vi "界面UI.vi"() -> ()   [LabVIEW 2016, in "德润DR803L超标留样.lvlib"]
uses:
  <vilib>/Utility/miscctls.llb/LVPointTypeDef.ctl
  <vilib>/Utility/config.llb/NI_LVConfig.lvlib
  <vilib>/ptbypt/NI_PtbyPt.lvlib
panel:
  in  "单步控制":bool
  in  "设置":bool
  out "采样器进程 2":T1(ring)
  out "单次采样量":u16
  out "留样模式":T2(ring)
  out "门状态":enum16{"门开", "门关"}(ring)
  out "报警状态":enum16{"无报警", "缺水报警"}(ring)
  out "仪器时间":timestamp format="%<%Y/%m/%d %H:%M:%S>T"
  out "当前瓶号":u16
  out "采样器状态":enum16{"停止", "运行"}(ring)
  out "采样器进程":i32(listbox)
  out "流程中":bool
  in  "停止流程":bool
  in  "启动流程":bool
  in  "修改门禁密码":bool
  in  "远程复位":bool
  in  "远程留样":bool
  out "Registers":u16[](array[numeric])
  in  "采样启动":bool
  in  "停止命令":bool
  in  "切换采样器状态":bool
  in  "时间校准":bool
  out "通讯":bool
  # "只在待机时启动有效"
  # "德润DR803L超标留样"
  # "只在待机时启动有效"
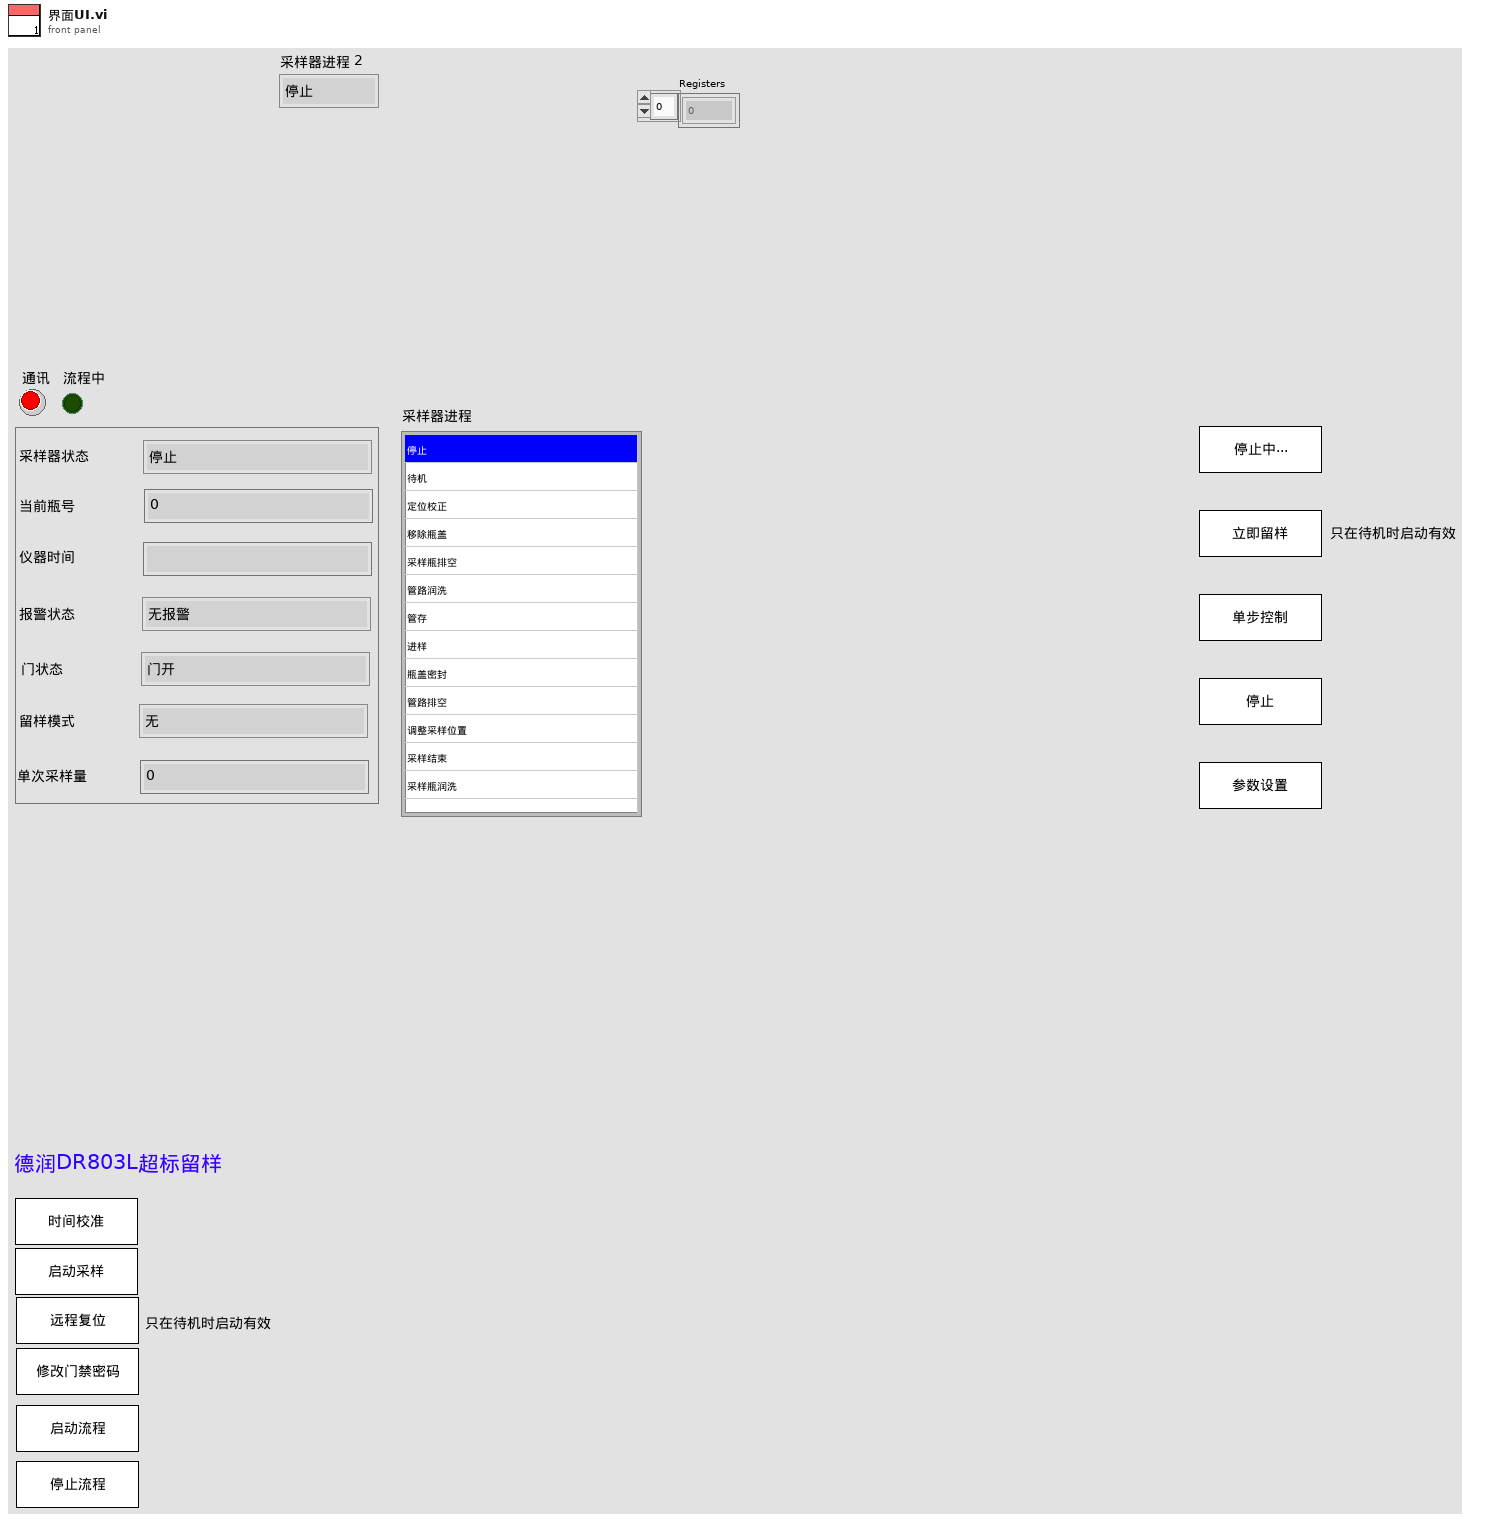
[diagram p1: front panel]
types:
  T1 = enum16{"停止", "待机", "定位校正", "移除瓶盖", "采样瓶排空", "管路润洗", "管存", "进样", "瓶盖密封", "管路排空", "调整采样位置", "采样结束", "采样瓶润洗", "瓶润洗排空"}
  T2 = enum16{"无", "定时留样", "时间等比例", "超标留样", "同步留样", "外控留样"}
  T3 = cluster{"STEP":enum16{"open", "read", "write", "write single", "close"}, "starting address":u16, "value":u16}
  T4 = typedef "LVPointTypeDef.ctl" = cluster{"Horizontal":i16, "Vertical":i16}
  T5 = typedef "NI_LVConfig.lvlib/Config Data RefNum.ctl" = refnum<k1>
  T6 = enum16{"open", "read", "write", "write single", "close"}
  T7 = typedef "LVDateTimeRec.ctl" = cluster{"秒数的小数部分":dbl, "秒":i32, "分":i32, "时":i32, "日":i32, "月":i32, "年":i32, "天数（周）":i32, "天数（年）":i32, "DST":i32}
  T8 = enum32{"Bad", "Idle", "Run top level", "Running"}
  T9 = cluster{"采样器状态":enum16{"停止", "运行"}, "当前留样瓶编号":u16, "报警状态":enum16{"无报警", "缺水报警"}, "超标信号":enum16{"无信号", "超标信号"}, "采样器进程":enum16{"停止", "待机", "定位校正", "移除瓶盖", "采样瓶排空", "管路润洗", "管存", "进样", "瓶盖密封", "管路排空", "调整采样位置", "采样结束", "采样瓶润洗", "瓶润洗排空"}, "版本号":string, "同步信号":enum16{"无信号", "同步信号"}, "外控信号":enum16{"无信号", "外控信号"}, "门状态":enum16{"门开", "门关"}, "当前瓶号":u16, "工作状态":enum16{"停止", "采样中"}, "留样模式":enum16{"无", "定时留样", "时间等比例", "超标留样", "同步留样", "外控留样"}, "立即留样":enum16{"无", "远程留样"}, "采样方式":enum16{"单采", "双重"}, "仪器时间":timestamp, "单次采样量":u16, "时间等比采样采样间隔":u16, "排空命令":u16, "远程复位":u16, "门禁密码":u16}
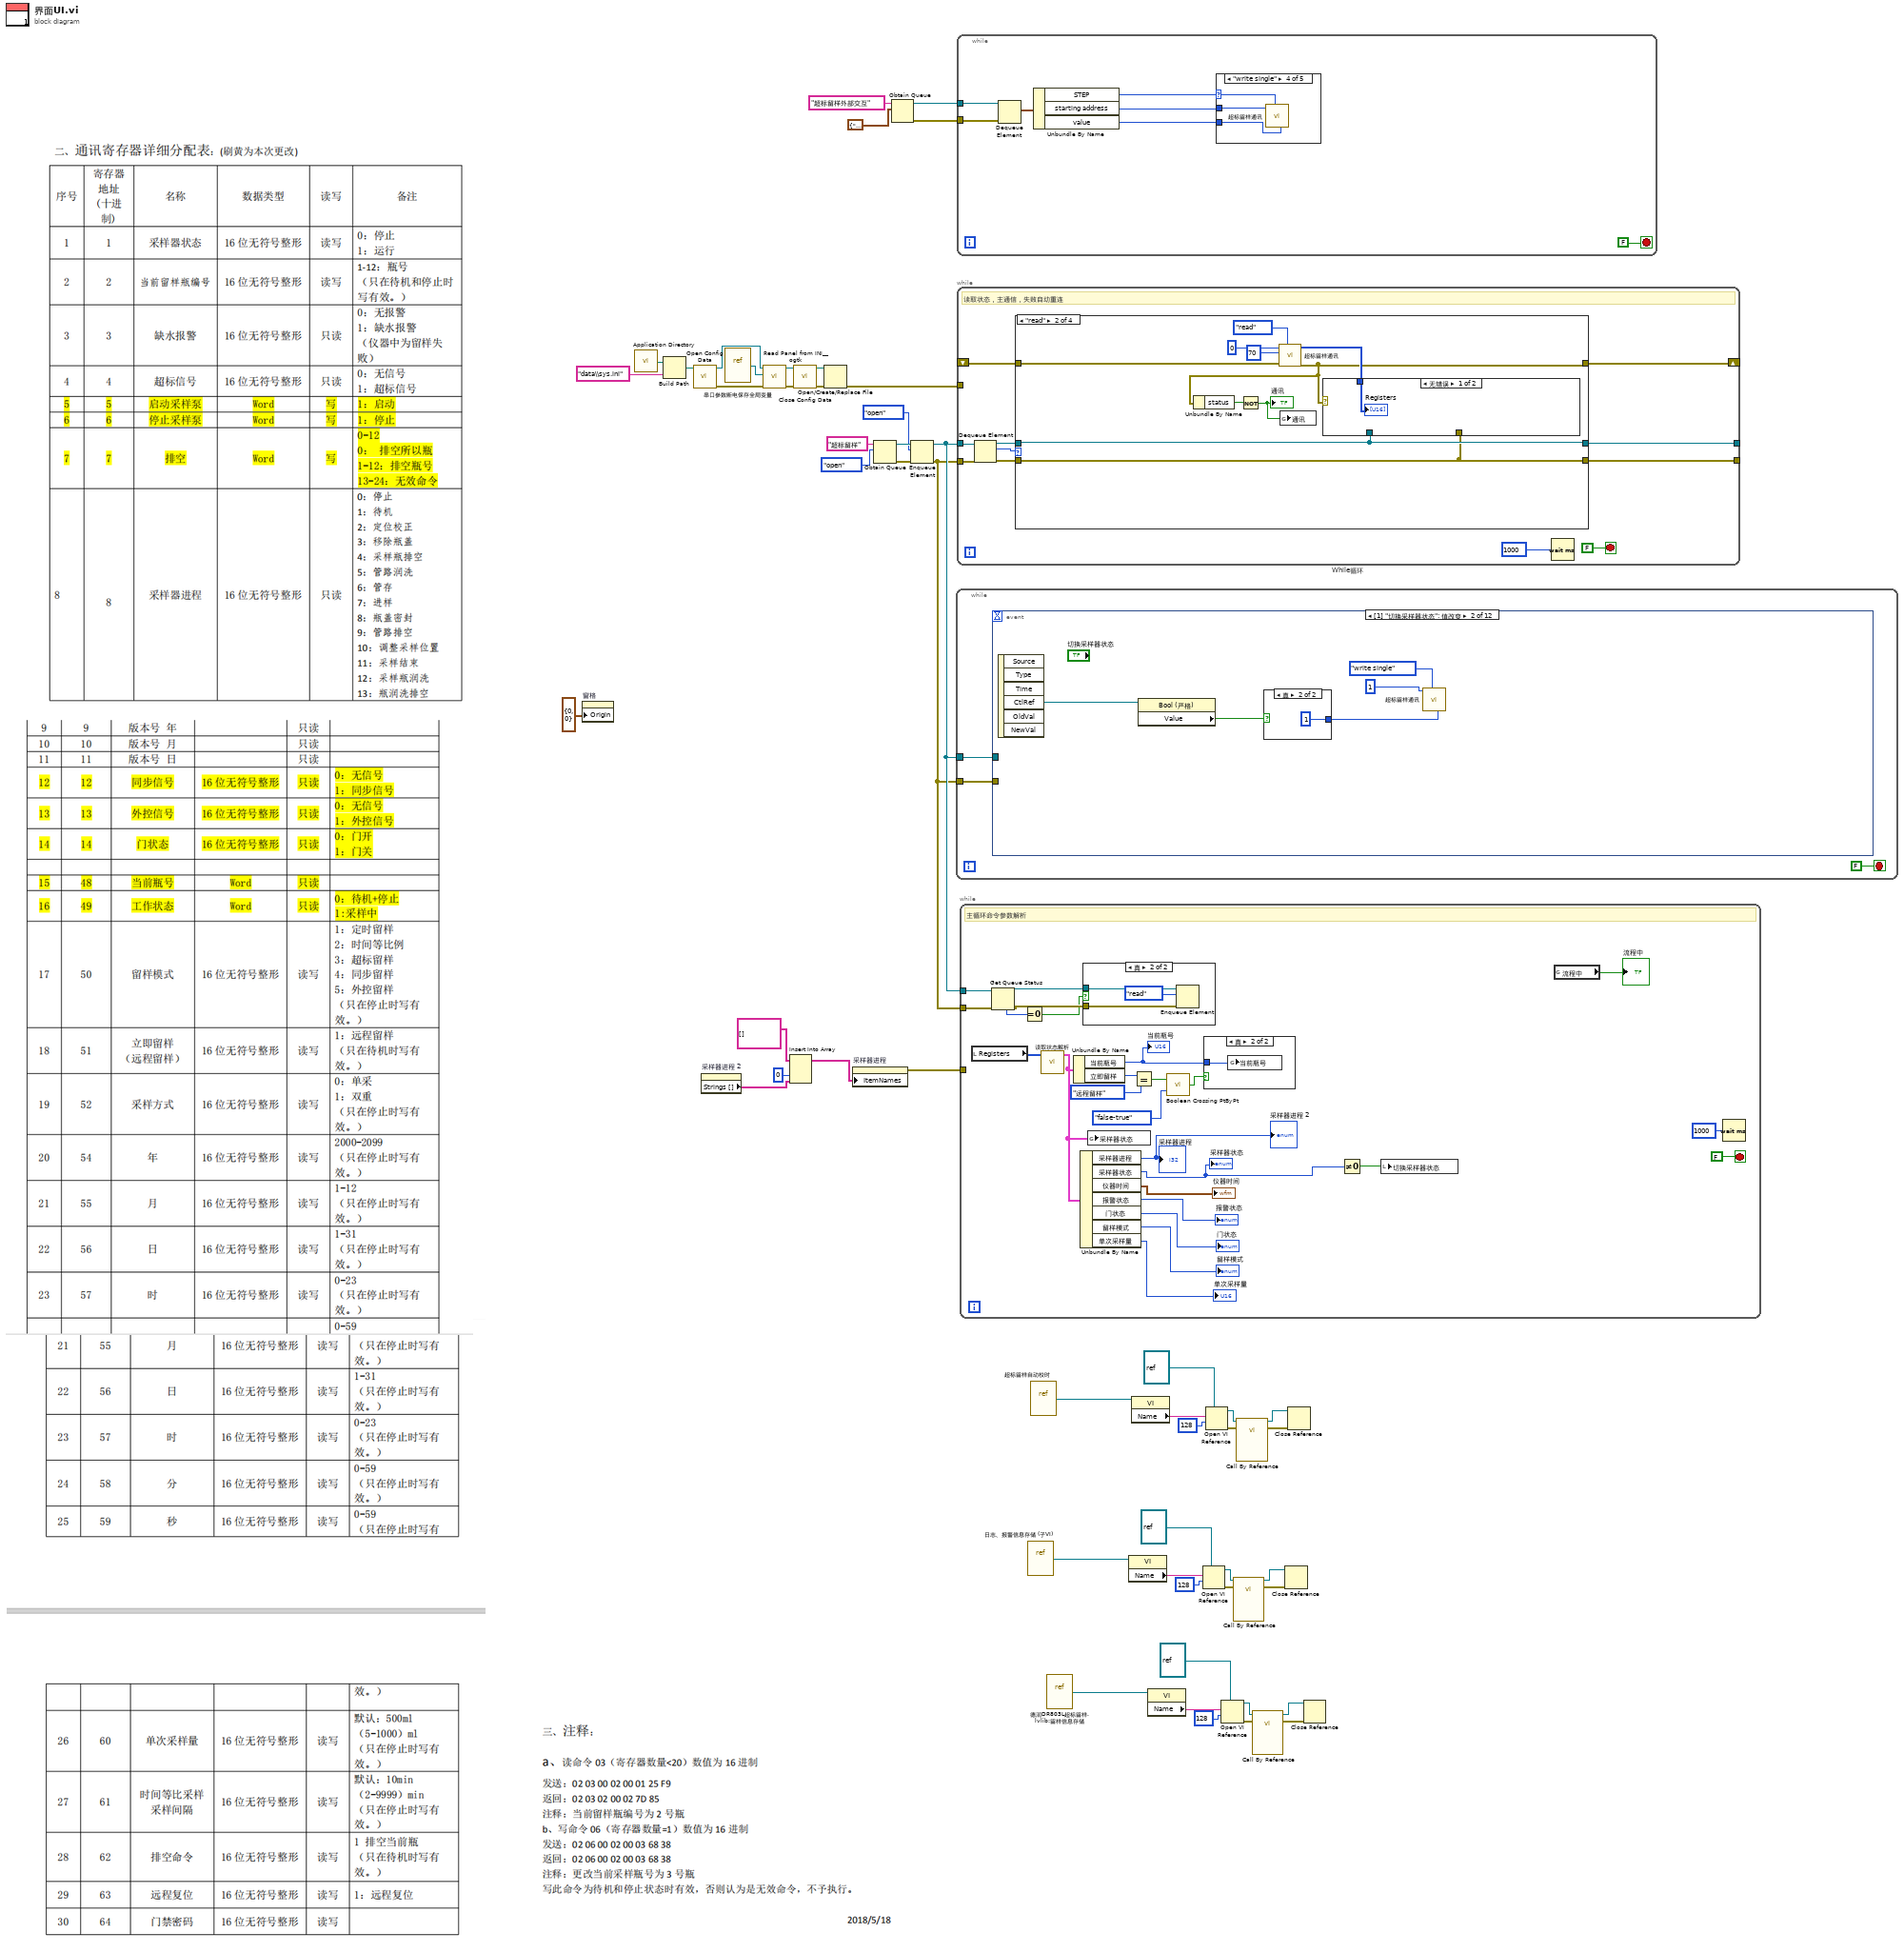
[diagram p0: block diagram]
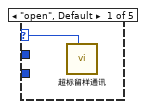
[diagram p2: hidden frame]
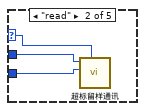
[diagram p3: hidden frame]
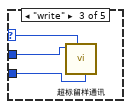
[diagram p4: hidden frame]
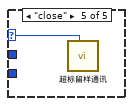
[diagram p5: hidden frame]
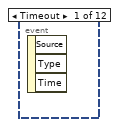
[diagram p6: hidden frame]
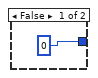
[diagram p7: hidden frame]
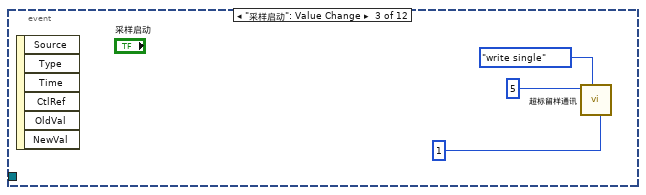
[diagram p8: hidden frame]
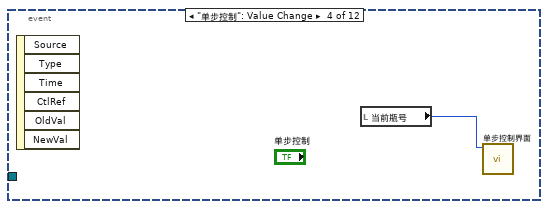
[diagram p9: hidden frame]
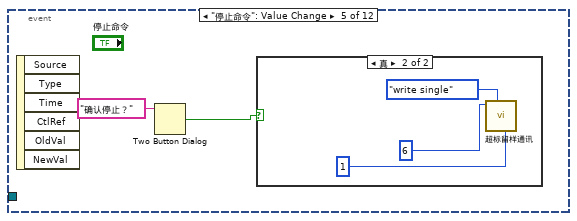
[diagram p10: hidden frame]
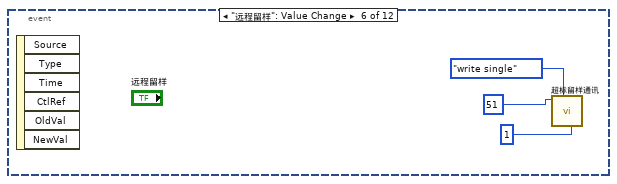
[diagram p12: hidden frame]
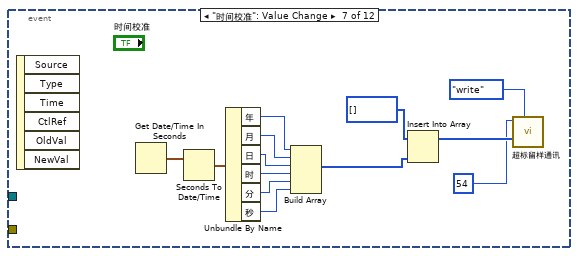
[diagram p13: hidden frame]
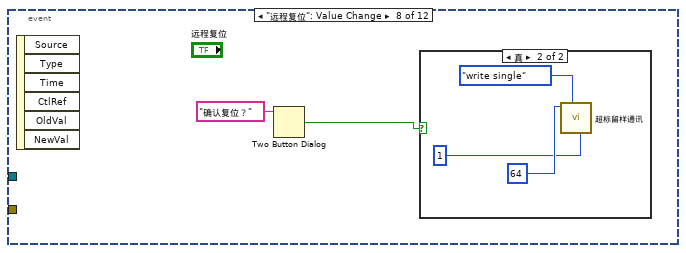
[diagram p14: hidden frame]
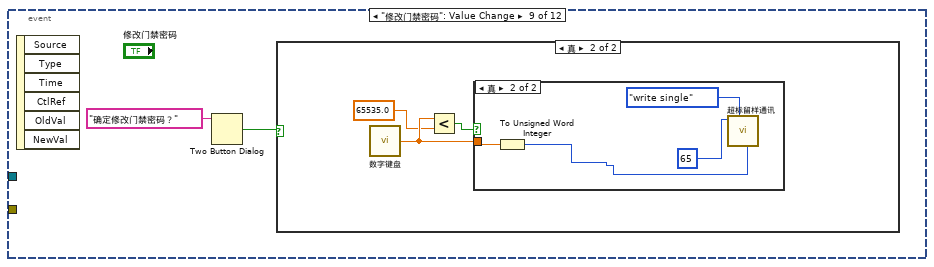
[diagram p16: hidden frame]
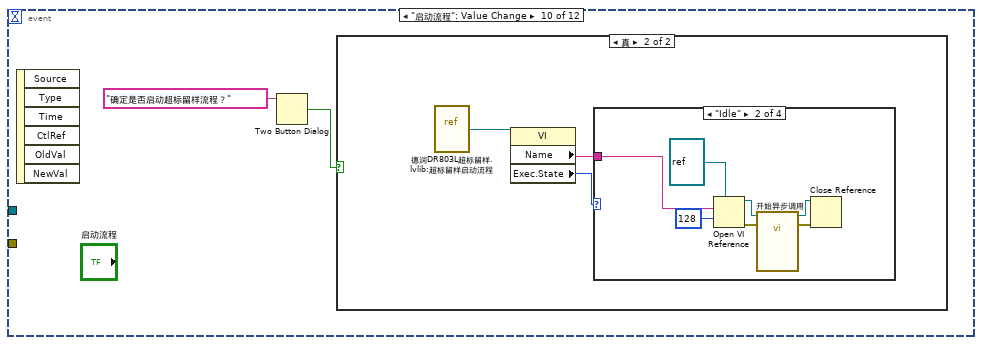
[diagram p19: hidden frame]
diagram:
  n1 = property on="窗格" class="Pane"("Origin"=T4 {"Horizontal"=0, "Vertical"=0} ("原点")) -> ()  [unwired: 2 in, 2 out]
  n2 = call <vilib>:"Application Directory.vi"() -> ("Application Directory"=w44:path)
  n3 = Build Path(base path=w44, name or relative path="data\\sys.ini" ("名称或相对路径")) -> (appended path=w42:path)
  n4 = call <vilib>:"Open Config Data.vi"("configuration file path"=w42) -> ("error out"=w38:errorcluster, "refnum"=w41:T5)  [unwired: 8 in, 1 out]
  n5 = property on="采样器进程 2" class="Enum (严格)"() -> ("Strings []"=w9:string[])  [unwired: 2 in, 2 out]
  n6 = vi-ref "串口参数断电保存全局变量.vi"() -> (w40:refnum<vi>)
  n7 = call <userlib>:"Read Panel from INI__ogtk.vi"("error in (no error)"=w38, "VI ref"=w40, "refnum"=w41) -> ("error out"=w37:errorcluster, "refnum out"=w39:T5)  [unwired: 7 in]
  n8 = Insert Into Array(array=string[][] [] ("字符串[]"), index (col)=0 ("禁用的索引 (列)"), new element=w9) -> (w11:string[][])  [unwired: 1 in]
  n9 = call <vilib>:"Close Config Data.vi"("error in (no error)"=w37, "refnum"=w39) -> ("error out"=w36:errorcluster, "file path"=w35:path)  [unwired: 8 in]
  n10 = Open/Create/Replace File(file path (use dialog)=w35, error in=w36) -> (error out=w34:errorcluster)  [unwired: 4 in, 2 out]
  n11 = property on="采样器进程" class="MCListbox (严格)"("ItemNames"=w11) -> (error out=w10:errorcluster)  [unwired: 2 in, 1 out]
  n12 = Obtain Queue(name (unnamed)="超标留样" ("名称（未命名）"), element data type=enum16{"open", "read", "write", "close"}."open") -> (queue out=w50:refnum<queue>, error out=w49:errorcluster)  [unwired: 3 in, 1 out]
  n13 = Obtain Queue(name (unnamed)="超标留样外部交互" ("名称（未命名）"), element data type=T3 {"STEP"=enum."write single", "starting address"=0, "value"=0}) -> (queue out=w31:refnum<queue>, error out=w30:errorcluster)  [unwired: 3 in, 1 out]
  n14 = Enqueue Element(queue=w50, element=enum16{"open", "read", "write", "close"}."open", error in (no error)=w49) -> (queue out=w47:refnum<queue>, error out=w46:errorcluster)  [unwired: 1 in, 1 out]
  n15 = while {
    tunnel: w47 -> [w54]
    tunnel: w46 -> [w53]
    stop <- FALSE stop-if-true
    n16 = event shown="[1] \"切换采样器状态\": 值改变" {
      selector: _ -> [_ _ _ _ _ _ _ _ _ _ _ _]
      dyn-events: _ -> [_ _ _ _ _ _ _ _ _ _ _ _]
      timeout: _ -> [_ _ _ _ _ _ _ _ _ _ _ _]
      tunnel: w54 -> [_ _ _ _ _ _ _ _ _ _ _ _]
      tunnel: w53 -> [_ _ _ _ _ _ _ _ _ _ _ _]
      event Timeout {
        n17 = event-data() -> ()  [unwired: 1 in, 3 out]
      }
      event "切换采样器状态": Value Change {
        n18 = event-data() -> ("CtlRef"=w60:refnum<vi>)  [unwired: 1 in, 5 out]
        n19 = property class="Bool (严格)"(reference=w60) -> ("Value"=w59:bool)  [unwired: 1 in, 2 out]
        n20 = case shown="真" w59 {
          tunnel: [u16 0 ("索引") u16 1 ("索引")] -> w56
          frame False {
          }
          frame True {
          }
        }
        n21 = call "超标留样通讯.vi"("value"=w56, "STEP"=T6."write single", "starting address"=1 ("索引")) -> ()  [unwired: 6 in, 3 out]
      }
      event "采样启动": Value Change {
        n22 = event-data() -> ()  [unwired: 1 in, 6 out]
        n23 = call "超标留样通讯.vi"("value"=u16 1 ("新元素/子数组"), "STEP"=T6."write single", "starting address"=5 ("索引")) -> ()  [unwired: 6 in, 3 out]
      }
      event "单步控制": Value Change {
        n24 = event-data() -> ()  [unwired: 1 in, 6 out]
        n25 = local read "当前瓶号"() -> (w66:u16)
        n26 = call "单步控制界面.vi"("当前瓶号"=w66) -> ()  [unwired: 11 in]
      }
      event "停止命令": Value Change {
        n27 = event-data() -> ()  [unwired: 1 in, 6 out]
        n28 = Two Button Dialog(message="确认停止？" ("消息")) -> (T button?=w67:bool)  [unwired: 2 in]
        n29 = case shown="真" w67 {
          frame False {
          }
          frame True {
            n30 = call "超标留样通讯.vi"("value"=u16 1 ("新元素/子数组"), "STEP"=T6."write single", "starting address"=6 ("索引")) -> ()  [unwired: 6 in, 3 out]
          }
        }
      }
      event "远程留样": Value Change {
        n31 = event-data() -> ()  [unwired: 1 in, 6 out]
        n32 = call "超标留样通讯.vi"("value"=u16 1 ("新元素/子数组"), "STEP"=T6."write single", "starting address"=51 ("索引")) -> ()  [unwired: 6 in, 3 out]
      }
      event "时间校准": Value Change {
        n33 = event-data() -> ()  [unwired: 1 in, 6 out]
        n34 = Get Date/Time In Seconds() -> (seconds since 1Jan1904=w87:timestamp)
        n35 = Seconds To Date/Time(time stamp (now)=w87) -> (date time rec=w86:T7)  [unwired: 1 in]
        n36 = Unbundle By Name(w86) -> ("年"=w83:i32, "月"=w82:i32, "日"=w81:i32, "时"=w80:i32, "分"=w79:i32, "秒"=w78:i32)
        n37 = Build Array(w83, w82, w81, w80, w79, w78) -> (w77:i32[])
        n38 = Insert Into Array(array=u16[] [] ("values"), new element=w77) -> (w84:u16[])  [unwired: 1 in]
        n39 = call "超标留样通讯.vi"("STEP"=T6."write", "values"=w84, "starting address"=54 ("索引")) -> ()  [unwired: 6 in, 3 out]
      }
      event "远程复位": Value Change {
        n40 = event-data() -> ()  [unwired: 1 in, 6 out]
        n41 = Two Button Dialog(message="确认复位？" ("消息")) -> (T button?=w88:bool)  [unwired: 2 in]
        n42 = case shown="真" w88 {
          frame False {
          }
          frame True {
            n43 = call "超标留样通讯.vi"("value"=u16 1 ("新元素/子数组"), "STEP"=T6."write single", "starting address"=64 ("索引")) -> ()  [unwired: 6 in, 3 out]
          }
        }
      }
      event "修改门禁密码": Value Change {
        n44 = event-data() -> ()  [unwired: 1 in, 6 out]
        n45 = Two Button Dialog(message="确定修改门禁密码？" ("消息")) -> (T button?=w93:bool)  [unwired: 2 in]
        n46 = case shown="真" w93 {
          frame False {
          }
          frame True {
            n47 = call "数字键盘.vi"() -> ("NewNumber"=w97:sgl)  [unwired: 1 in]
            n48 = Less?(x=w97, y=sgl 65535.0) -> (x < y?=w95:bool)
            n49 = case shown="真" w95 {
              tunnel: w97 -> [_ w101]
              frame False {
              }
              frame True {
                n50 = To Unsigned Word Integer(number=w101) -> (unsigned 16bit integer=w98:u16)
                n51 = call "超标留样通讯.vi"("value"=w98, "STEP"=T6."write single", "starting address"=65 ("索引")) -> ()  [unwired: 6 in, 3 out]
              }
            }
          }
        }
      }
      event "启动流程": Value Change {
        n52 = event-data() -> ()  [unwired: 1 in, 6 out]
        n53 = Two Button Dialog(message="确定是否启动超标留样流程？" ("消息")) -> (T button?=w102:bool)  [unwired: 2 in]
        n54 = case shown="真" w102 {
          frame False {
          }
          frame True {
            n55 = vi-ref "德润DR803L超标留样.lvlib:超标留样启动流程.vi"() -> (w104:refnum<vi>)
            n56 = property class="VI"(reference=w104) -> ("Name"=w105:string, "Exec.State"=w106:T8)  [unwired: 1 in, 2 out]
            n57 = case shown="\"Idle\"" w106 {
              tunnel: w105 -> [_ w109 _ _]
              frame "Bad", Default {
              }
              frame "Idle" {
                n58 = Open VI Reference(type specifier VI Refnum (for type only)=refnum<vi> refnum ("类型说明符VI引用句柄（仅用于类型）"), vi path=w109, options=128 ("选项")) -> (vi reference=w113:refnum<vi>, error out=w108:errorcluster)  [unwired: 3 in]
                n59 = call-by-ref "开始异步调用"(reference=w113, error in=w108) -> (reference out=w112:refnum<vi>, error out=w107:errorcluster)  [unwired: 12 in]
                n60 = Close Reference(reference=w112, error in (no error)=w107) -> ()  [unwired: 1 out]
              }
              frame "Run top level" {
              }
              frame "Running" {
              }
            }
          }
        }
      }
      event "停止流程": Value Change {
        n61 = event-data() -> ()  [unwired: 1 in, 6 out]
        n62 = Two Button Dialog(message="确定是否停止超标留样流程并排空当前瓶？" ("消息")) -> (T button?=w114:bool)  [unwired: 2 in]
        n63 = case shown="真" w114 {
          frame False {
          }
          frame True {
            n64 = Obtain Notifier(name (unnamed)="超标留样流程" ("名称（未命名）"), notification data type=FALSE ("采样完成")) -> (notifier out=w127:refnum<notifier>, error out=w126:errorcluster)  [unwired: 2 in, 1 out]
            n65 = Send Notification(notification=TRUE ("通知"), notifier=w127, error in (no error)=w126) -> (notifier out=w124:refnum<notifier>, error out=w123:errorcluster)
            n66 = call "超标留样通讯.vi"("value"=u16 1 ("新元素/子数组"), "STEP"=T6."write single", "starting address"=6 ("索引")) -> ("error out"=w116:errorcluster)  [unwired: 6 in, 2 out]
            n67 = Release Notifier(notifier=w124, error in (no error)=w123) -> ()  [unwired: 1 in, 3 out]
            n68 = call "超标留样通讯.vi"("value"=u16 1 ("新元素/子数组"), "STEP"=T6."write single", "Error in"=w116, "starting address"=63 ("索引")) -> ()  [unwired: 5 in, 3 out]
          }
        }
      }
      event "设置": Value Change {
        n69 = event-data() -> ()  [unwired: 1 in, 6 out]
        n70 = global read "超标留样全局.vi" "采样器状态"() -> (w134:T9)
        n71 = Unbundle By Name(w134) -> ("留样模式"=w133:T2, "采样方式"=w132:enum16{"单采", "双重"}, "单次采样量"=w131:u16, "时间等比采样采样间隔"=w130:u16)
        n72 = call "参数设置对画框.vi"("时间等比采样"=w130, "单次采样量"=w131, "采样方式"=w132, "留样模式"=w133) -> ()  [unwired: 8 in]
      }
    }
  }
  n73 = while {
    tunnel: w31 -> [w140]
    tunnel: w30 -> [w139]
    stop <- FALSE stop-if-true
    n74 = Dequeue Element(queue=w140, error in (no error)=w139) -> (element=w138:T3)  [unwired: 1 in, 3 out]
    n75 = Unbundle By Name(w138) -> ("STEP"=w137:T6, "starting address"=w136:u16, "value"=w135:u16)
    n76 = case shown="\"write single\"" w137 {
      selector: w137 -> [w142 w145 w148 w151 w152]
      tunnel: w136 -> [_ w144 w147 w150 _]
      tunnel: w135 -> [_ w143 w146 w149 _]
      frame "open", Default {
        n77 = call "超标留样通讯.vi"("STEP"=w142) -> ()  [unwired: 8 in, 3 out]
      }
      frame "read" {
        n78 = call "超标留样通讯.vi"("STEP"=w145, "quantity"=w143, "starting address"=w144) -> ()  [unwired: 6 in, 3 out]
      }
      frame "write" {
        n79 = call "超标留样通讯.vi"("value"=w146, "STEP"=w148, "starting address"=w147) -> ()  [unwired: 6 in, 3 out]
      }
      frame "write single" {
        n80 = call "超标留样通讯.vi"("value"=w149, "STEP"=w151, "starting address"=w150) -> ()  [unwired: 6 in, 3 out]
      }
      frame "close" {
        n81 = call "超标留样通讯.vi"("STEP"=w152) -> ()  [unwired: 8 in, 3 out]
      }
    }
  }
  n82 = while "While循环" {
    tunnel: w47 -> [w154]
    tunnel: w46 -> [w153]
    tunnel: [w158] -> _
    tunnel: [w157] -> _
    shift-right: [w155] -> _
    shift-left: _ -> [w156]
    tunnel: w34 -> [_]
    stop <- FALSE stop-if-true
    # "读取状态，主通信，失败自动重连"
    n83 = Dequeue Element(queue=w154, error in (no error)=w153) -> (queue out=w160:refnum<queue>, element=w161:enum16{"open", "read", "write", "close"}, error out=w159:errorcluster)  [unwired: 1 in, 1 out]
    n84 = case shown="\"read\"" w161 {
      tunnel: [w169 w171 w189 w198] -> w155
      tunnel: w160 -> [w168 w174 w188 w201]
      tunnel: w159 -> [w167 w173 w187 w200]
      tunnel: [w168 w174 w188 w201] -> w158
      tunnel: [w167 w173 w187 w200] -> w157
      tunnel: w156 -> [w166 w179 w191 w202]
      frame "open", Default {
        n85 = call "超标留样通讯.vi"("STEP"=T6."open", "Error in"=w166) -> ("error out"=w169:errorcluster, "MB session in"=w165:refnum<class "MB_Master.lvclass">)  [unwired: 7 in, 1 out]
        n86 = global write "串口参数断电保存全局变量.vi" "MB session in"(w165) -> ()
      }
      frame "read" {
        n87 = call "超标留样通讯.vi"("STEP"=T6."read", "Error in"=w179, "quantity"=u16 70, "starting address"=u16 0) -> ("error out"=w171:errorcluster, "Registers"=w176:u16[])  [unwired: 5 in, 1 out]
        n88 = Unbundle By Name(w171) -> ("status"=w172:bool)
        n89 = Not(x=w172) -> (.not. x?=w170:bool)
        "通讯" <- w170
        n90 = global write "超标留样全局.vi" "通讯"(w170) -> ()
        n91 = case shown="无错误" w171 {
          tunnel: w176 -> [w180 _]
          tunnel: w174 -> [_ w185]
          tunnel: w173 -> [_ w184]
          frame No Error {
            "Registers" <- w180
          }
          frame Error {
            n92 = Enqueue Element(queue=w185, element=enum16{"open", "read", "write", "close"}."close" ("元素"), error in (no error)=w184) -> (queue out=w183:refnum<queue>, error out=w182:errorcluster)  [unwired: 1 in, 1 out]
            n93 = Enqueue Element(queue=w183, element=enum16{"open", "read", "write", "close"}."open" ("元素"), error in (no error)=w182) -> ()  [unwired: 1 in, 3 out]
          }
        }
      }
      frame "write" {
        n94 = call "超标留样通讯.vi"("STEP"=T6."write single", "Error in"=w191) -> ("error out"=w189:errorcluster)  [unwired: 7 in, 2 out]
        n95 = case shown="错误" w189 {
          tunnel: w188 -> [_ w193]
          tunnel: w187 -> [_ w192]
          frame No Error {
          }
          frame Error {
            n96 = Enqueue Element(queue=w193, element=enum16{"open", "read", "write", "close"}."close" ("元素"), error in (no error)=w192) -> (queue out=w196:refnum<queue>, error out=w195:errorcluster)  [unwired: 1 in, 1 out]
            n97 = Enqueue Element(queue=w196, element=enum16{"open", "read", "write", "close"}."open" ("元素"), error in (no error)=w195) -> ()  [unwired: 1 in, 3 out]
          }
        }
      }
      frame "close" {
        n98 = call "超标留样通讯.vi"("STEP"=T6."close", "Error in"=w202) -> ("error out"=w198:errorcluster)  [unwired: 7 in, 2 out]
      }
    }
    n99 = Wait (ms)(milliseconds to wait=u32 1000 ("等待时间（毫秒）")) -> ()  [unwired: 1 out]
  }
  n100 = while {
    tunnel: w47 -> [w225]
    tunnel: w46 -> [w224]
    tunnel: w10 -> [_]
    stop <- FALSE stop-if-true
    # "主循环命令参数解析"
    n101 = local read "Registers"() -> (w219:u16[])
    n102 = Get Queue Status(queue=w225, error in (no error)=w224) -> (queue out=w222:refnum<queue>, error out=w221:errorcluster, # elements in queue=w223:i32)  [unwired: 1 in, 5 out]
    n103 = Equal To 0?(x=w223) -> (x = 0?=w220:bool)
    n104 = call "读取状态解析.vi"("Registers"=w219) -> ("采样器状态"=w212:T9)  [unwired: 9 in, 1 out]
    n105 = Unbundle By Name(w212) -> ("当前瓶号"=w211:u16, "立即留样"=w218:enum16{"无", "远程留样"})
    "当前瓶号" <- w211
    n106 = Unbundle By Name(w212) -> ("采样器进程"=→"采样器进程" →"采样器进程 2":T1, "采样器状态"=w204:enum16{"停止", "运行"}, "仪器时间"=→"仪器时间":timestamp, "报警状态"=→"报警状态":enum16{"无报警", "缺水报警"}, "门状态"=→"门状态":enum16{"门开", "门关"}, "留样模式"=→"留样模式":T2, "单次采样量"=→"单次采样量":u16)
    "采样器状态" <- w204
    n107 = case shown="真" w220 {
      tunnel: w222 -> [_ w230]
      tunnel: w221 -> [_ w229]
      frame False {
      }
      frame True {
        n108 = Enqueue Element(queue=w230, element=enum16{"open", "read", "write", "close"}."read" ("元素"), error in (no error)=w229) -> ()  [unwired: 1 in, 3 out]
      }
    }
    n109 = global write "超标留样全局.vi" "采样器状态"(w212) -> ()
    n110 = Equal?(x=w218, y=enum16{"无", "远程留样"}."远程留样") -> (x = y?=w217:bool)
    n111 = call <vilib>:"Boolean Crossing PtByPt.vi"("direction"=enum16{"either", "false-true", "true-false"}."false-true", "input"=w217) -> ("crossing"=w215:bool)  [unwired: 1 in]
    n112 = case shown="真" w215 {
      tunnel: w211 -> [_ w228]
      frame False {
      }
      frame True {
        n113 = global write "超标留样全局.vi" "当前瓶号"(w228) -> ()
      }
    }
    n114 = Not Equal To 0?(x=w204) -> (x != 0?=w203:bool)
    n115 = local write "切换采样器状态"(w203) -> ()
    n116 = global read "串口参数断电保存全局变量.vi" "流程中"() -> (→"流程中":bool)
    n117 = Wait (ms)(milliseconds to wait=u32 1000 ("等待时间（毫秒）")) -> ()  [unwired: 1 out]
  }
  n118 = vi-ref "日志、报警信息存储 (子VI).vi"() -> (w22:refnum<vi>)
  n119 = vi-ref "超标留样自动校时.vi"() -> (w21:refnum<vi>)
  n120 = vi-ref "德润DR803L超标留样.lvlib:留样信息存储.vi"() -> (w8:refnum<vi>)
  n121 = property class="VI"(reference=w22) -> ("Name"=w23:string)  [unwired: 1 in, 2 out]
  n122 = property class="VI"(reference=w21) -> ("Name"=w20:string)  [unwired: 1 in, 2 out]
  n123 = property class="VI"(reference=w8) -> ("Name"=w7:string)  [unwired: 1 in, 2 out]
  n124 = Open VI Reference(type specifier VI Refnum (for type only)=refnum<vi> refnum, vi path=w23, options=128 ("选项")) -> (vi reference=w25:refnum<vi>, error out=w27:errorcluster)  [unwired: 3 in]
  n125 = Open VI Reference(type specifier VI Refnum (for type only)=refnum<vi> refnum, vi path=w20, options=128 ("选项")) -> (vi reference=w18:refnum<vi>, error out=w16:errorcluster)  [unwired: 3 in]
  n126 = Open VI Reference(type specifier VI Refnum (for type only)=refnum<vi> refnum, vi path=w7, options=128 ("选项")) -> (vi reference=w5:refnum<vi>, error out=w3:errorcluster)  [unwired: 3 in]
  n127 = call-by-ref "?"(reference=w25, error in=w27) -> (reference out=w29:refnum<vi>, error out=w28:errorcluster)  [unwired: 12 in]
  n128 = call-by-ref "?"(reference=w18, error in=w16) -> (reference out=w14:refnum<vi>, error out=w15:errorcluster)  [unwired: 12 in]
  n129 = call-by-ref "?"(reference=w5, error in=w3) -> (reference out=w1:refnum<vi>, error out=w2:errorcluster)  [unwired: 12 in]
  n130 = Close Reference(reference=w29, error in (no error)=w28) -> ()  [unwired: 1 out]
  n131 = Close Reference(reference=w14, error in (no error)=w15) -> ()  [unwired: 1 out]
  n132 = Close Reference(reference=w1, error in (no error)=w2) -> ()  [unwired: 1 out]
